vi "CollectCopyrightNotices.vi"() -> ()   [LabVIEW 2020]
uses:
  abd7129a-8e98-49aa-842b-ff99d9e25c9b.vi
panel:
  in  "Folder Path":path
  out "Missing Entires":string[](array[string]) caption="Missing Entires - Anything other than \"pkgconf or vcpkg-*\" needs fixing"
  out "error out":errorcluster
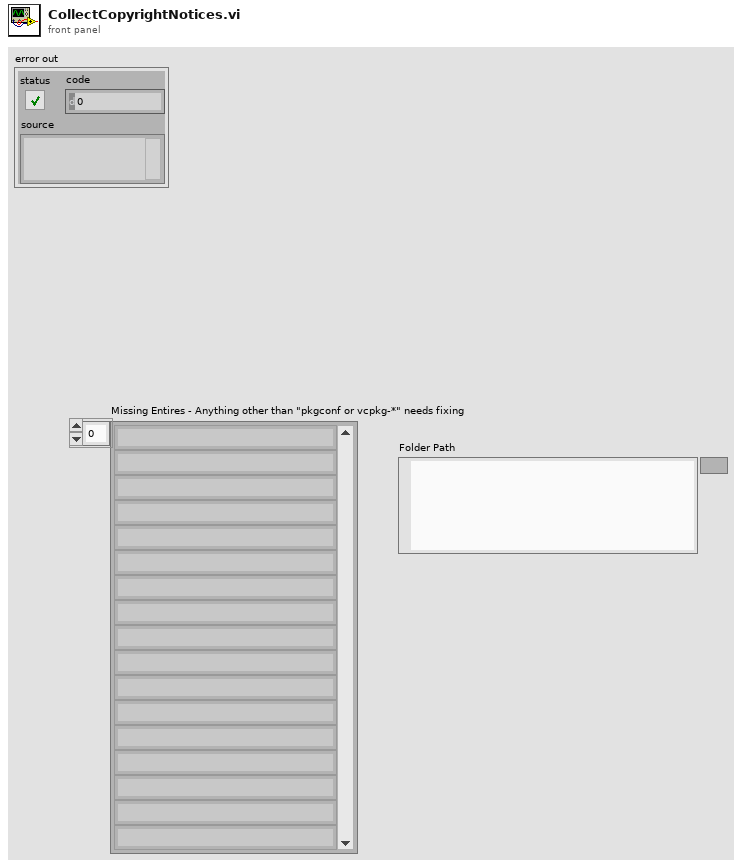
[diagram p1: front panel]
types:
  T1 = enum16{"open", "replace", "create", "open or create", "replace or create", "replace or create with confirmation"}
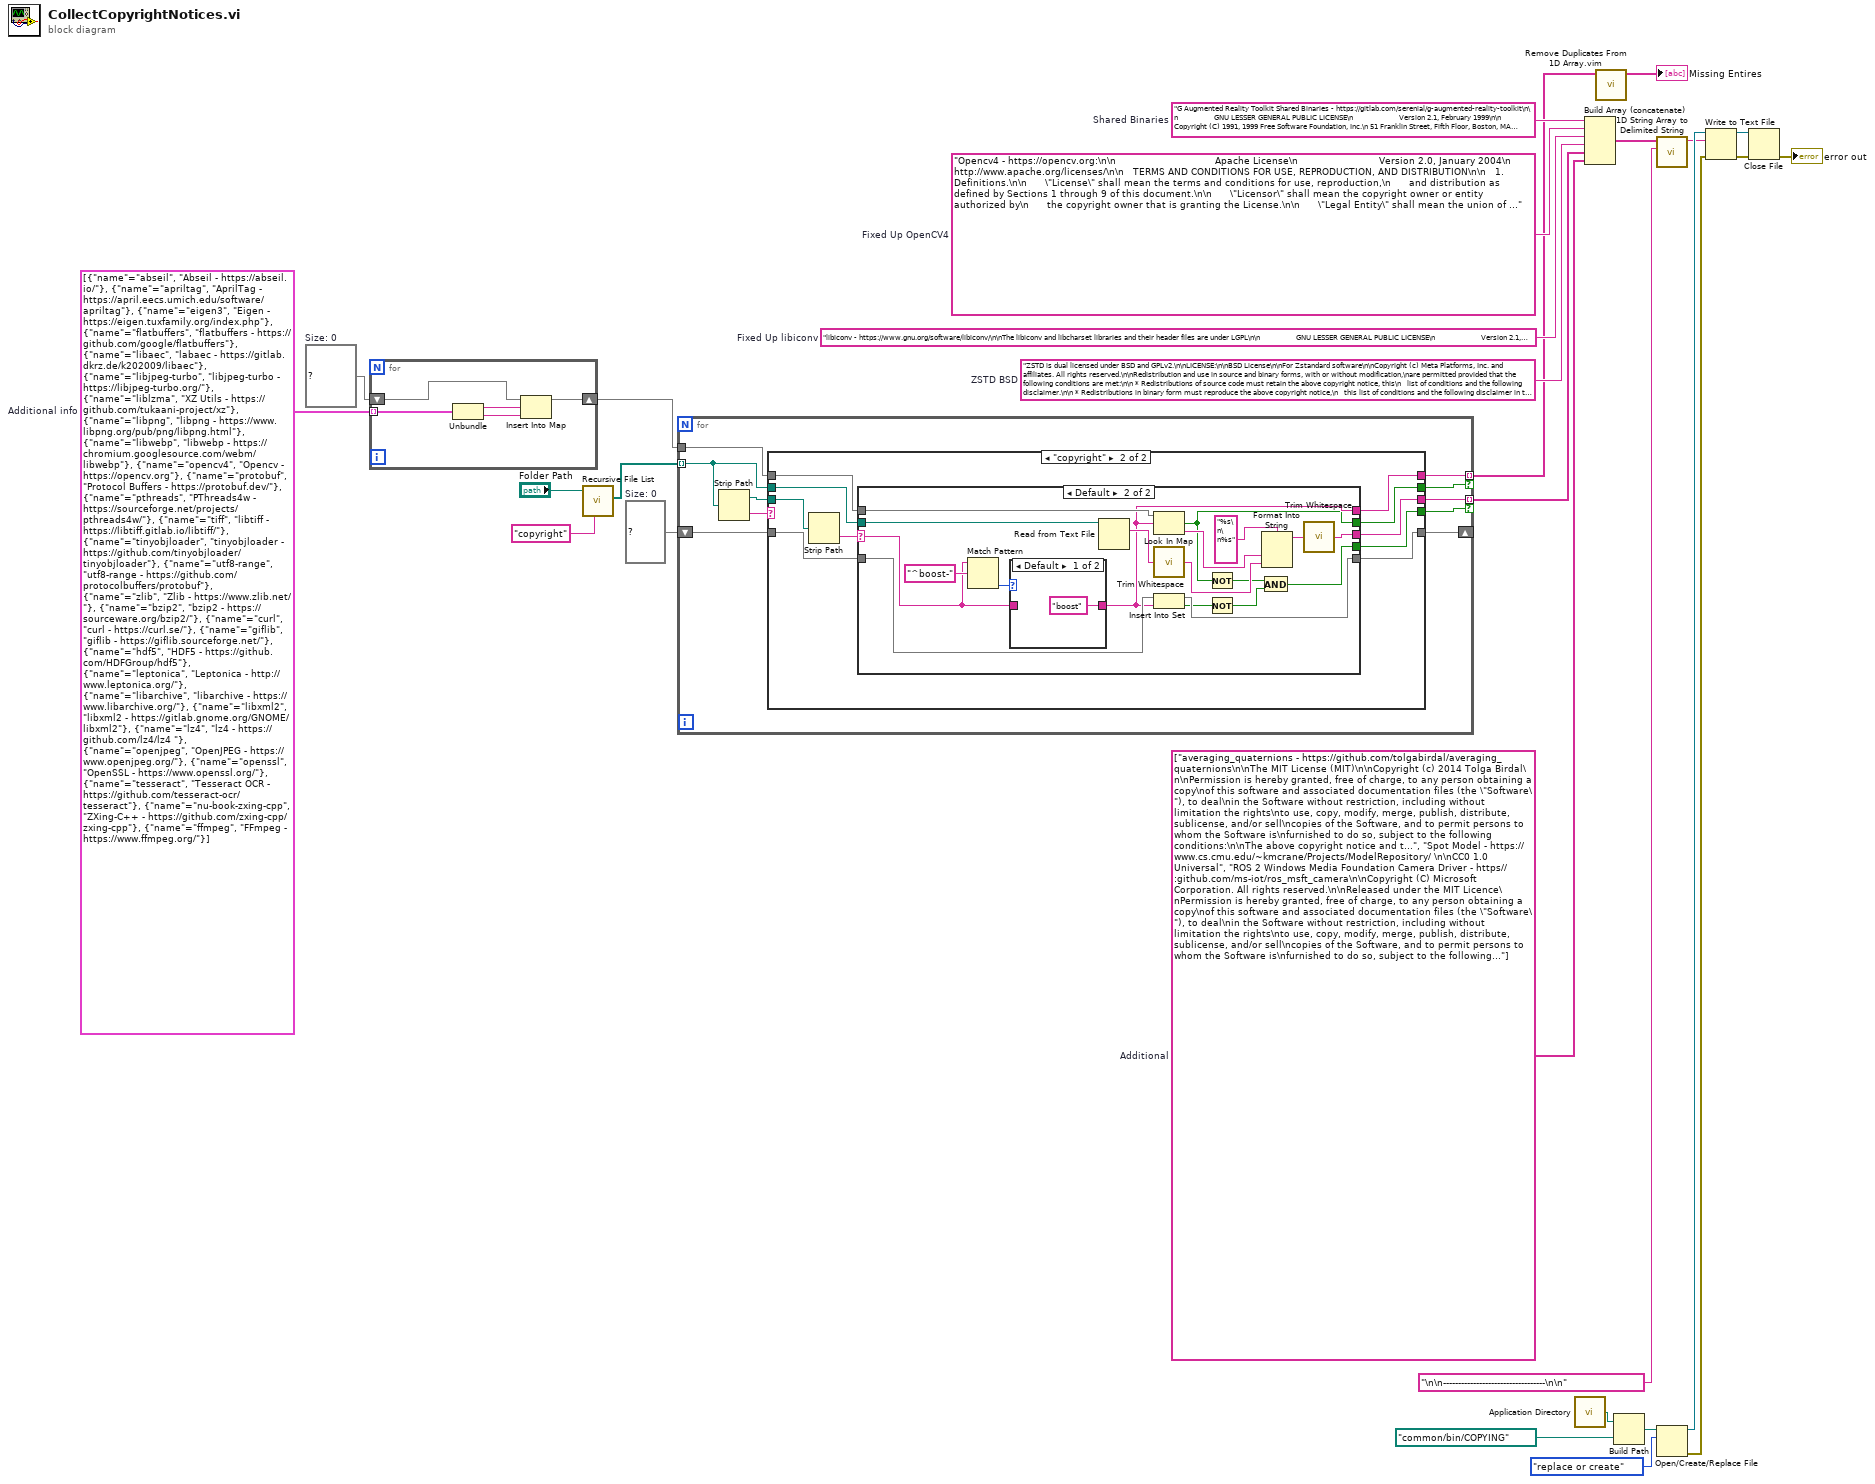
[diagram p0: block diagram]
diagram:
  w4 = "G Augmented Reality Toolkit Shared Binaries - https://gitlab.com/serenial/g-augmented-reality-toolkit\n\n                  GNU LESSER GENERAL PUBLIC LICENSE\n                       Version 2.1, February 1999\n\n Copyright (C) 1991, 1999 Free Software Foundation, Inc.\n 51 Franklin Street, Fifth Floor, Boston, MA  02110-1301  USA\n Everyone is permitted to copy and distribute verbatim copies\n of this license document, but changing it is not allowed.\n\n[This is the first released version of the Lesser GPL.  It also counts\n as the successor of the GNU Library Public License, version 2, hence\n the version number 2.1.]\n\n                            Preamble\n\n  The licenses for most software are designed to take away your\nfreedom to share and change it.  By contrast, the GNU General Public\nLicenses are intended to guarantee your freedom to share and change\nfree software--to make sure the software is free for all its users.\n\n  This license, the Lesser General Public License, applies to some\nspecially designated software packages--typically libraries--of the\nFree Software Foundation and other authors who decide to use it.  You\ncan use it too, but we suggest you first think carefully about whether\nthis license or the ordinary General Public License is the better\nstrategy to use in any particular case, based on the explanations below.\n\n  When we speak of free software, we are referring to freedom of use,\nnot price.  Our General Public Licenses are designed to make sure that\nyou have the freedom to distribute copies of free software (and charge\nfor this service if you wish); that you receive source code or can get\nit if you want it; that you can change the software and use pieces of\nit in new free programs; and that you are informed that you can do\nthese things.\n\n  To protect your rights, we need to make restrictions that forbid\ndistributors to deny you these rights or to ask you to surrender these\nrights.  These restrictions translate to certain responsibilities for\nyou if you distribute copies of the library or if you modify it.\n\n  For example, if you distribute copies of the library, whether gratis\nor for a fee, you must give the recipients all the rights that we gave\nyou.  You must make sure that they, too, receive or can get the source\ncode.  If you link other code with the library, you must provide\ncomplete object files to the recipients, so that they can relink them\nwith the library after making changes to the library and recompiling\nit.  And you must show them these terms so they know their rights.\n\n  We protect your rights with a two-step method: (1) we copyright the\nlibrary, and (2) we offer you this license, which gives you legal\npermission to copy, distribute and/or modify the library.\n\n  To protect each distributor, we want to make it very clear that\nthere is no warranty for the free library.  Also, if the library is\nmodified by someone else and passed on, the recipients should know\nthat what they have is not the original version, so that the original\nauthor's reputation will not be affected by problems that might be\nintroduced by others.\n\n  Finally, software patents pose a constant threat to the existence of\nany free program.  We wish to make sure that a company cannot\neffectively restrict the users of a free program by obtaining a\nrestrictive license from a patent holder.  Therefore, we insist that\nany patent license obtained for a version of the library must be\nconsistent with the full freedom of use specified in this license.\n\n  Most GNU software, including some libraries, is covered by the\nordinary GNU General Public License.  This license, the GNU Lesser\nGeneral Public License, applies to certain designated libraries, and\nis quite different from the ordinary General Public License.  We use\nthis license for certain libraries in order to permit linking those\nlibraries into non-free programs.\n\n  When a program is linked with a library, whether statically or using\na shared library, the combination of the two is legally speaking a\ncombined work, a derivative of the original library.  The ordinary\nGeneral Public License therefore permits such linking only if the\nentire combination fits its criteria of freedom.  The Lesser General\nPublic License permits more lax criteria for linking other code with\nthe library.\n\n  We call this license the \"Lesser\" General Public License because it\ndoes Less to protect the user's freedom than the ordinary General\nPublic License.  It also provides other free software developers Less\nof an advantage over competing non-free programs.  These disadvantages\nare the reason we use the ordinary General Public License for many\nlibraries.  However, the Lesser license provides advantages in certain\nspecial circumstances.\n\n  For example, on rare occasions, there may be a special need to\nencourage the widest possible use of a certain library, so that it becomes\na de-facto standard.  To achieve this, non-free programs must be\nallowed to use the library.  A more frequent case is that a free\nlibrary does the same job as widely used non-free libraries.  In this\ncase, there is little to gain by limiting the free library to free\nsoftware only, so we use the Lesser General Public License.\n\n  In other cases, permission to use a particular library in non-free\nprograms enables a greater number of people to use a large body of\nfree software.  For example, permission to use the GNU C Library in\nnon-free programs enables many more people to use the whole GNU\noperating system, as well as its variant, the GNU/Linux operating\nsystem.\n\n  Although the Lesser General Public License is Less protective of the\nusers' freedom, it does ensure that the user of a program that is\nlinked with the Library has the freedom and the wherewithal to run\nthat program using a modified version of the Library.\n\n  The precise terms and conditions for copying, distribution and\nmodification follow.  Pay close attention to the difference between a\n\"work based on the library\" and a \"work that uses the library\".  The\nformer contains code derived from the library, whereas the latter must\nbe combined with the library in order to run.\n\n                  GNU LESSER GENERAL PUBLIC LICENSE\n   TERMS AND CONDITIONS FOR COPYING, DISTRIBUTION AND MODIFICATION\n\n  0. This License Agreement applies to any software library or other\nprogram which contains a notice placed by the copyright holder or\nother authorized party saying it may be distributed under the terms of\nthis Lesser General Public License (also called \"this License\").\nEach licensee is addressed as \"you\".\n\n  A \"library\" means a collection of software functions and/or data\nprepared so as to be conveniently linked with application programs\n(which use some of those functions and data) to form executables.\n\n  The \"Library\", below, refers to any such software library or work\nwhich has been distributed under these terms.  A \"work based on the\nLibrary\" means either the Library or any derivative work under\ncopyright law: that is to say, a work containing the Library or a\nportion of it, either verbatim or with modifications and/or translated\nstraightforwardly into another language.  (Hereinafter, translation is\nincluded without limitation in the term \"modification\".)\n\n  \"Source code\" for a work means the preferred form of the work for\nmaking modifications to it.  For a library, complete source code means\nall the source code for all modules it contains, plus any associated\ninterface definition files, plus the scripts used to control compilation\nand installation of the library.\n\n  Activities other than copying, distribution and modification are not\ncovered by this License; they are outside its scope.  The act of\nrunning a program using the Library is not restricted, and output from\nsuch a program is covered only if its contents constitute a work based\non the Library (independent of the use of the Library in a tool for\nwriting it).  Whether that is true depends on what the Library does\nand what the program that uses the Library does.\n\n  1. You may copy and distribute verbatim copies of the Library's\ncomplete source code as you receive it, in any medium, provided that\nyou conspicuously and appropriately publish on each copy an\nappropriate copyright notice and disclaimer of warranty; keep intact\nall the notices that refer to this License and to the absence of any\nwarranty; and distribute a copy of this License along with the\nLibrary.\n\n  You may charge a fee for the physical act of transferring a copy,\nand you may at your option offer warranty protection in exchange for a\nfee.\n\n  2. You may modify your copy or copies of the Library or any portion\nof it, thus forming a work based on the Library, and copy and\ndistribute such modifications or work under the terms of Section 1\nabove, provided that you also meet all of these conditions:\n\n    a) The modified work must itself be a software library.\n\n    b) You must cause the files modified to carry prominent notices\n    stating that you changed the files and the date of any change.\n\n    c) You must cause the whole of the work to be licensed at no\n    charge to all third parties under the terms of this License.\n\n    d) If a facility in the modified Library refers to a function or a\n    table of data to be supplied by an application program that uses\n    the facility, other than as an argument passed when the facility\n    is invoked, then you must make a good faith effort to ensure that,\n    in the event an application does not supply such function or\n    table, the facility still operates, and performs whatever part of\n    its purpose remains meaningful.\n\n    (For example, a function in a library to compute square roots has\n    a purpose that is entirely well-defined independent of the\n    application.  Therefore, Subsection 2d requires that any\n    application-supplied function or table used by this function must\n    be optional: if the application does not supply it, the square\n    root function must still compute square roots.)\n\nThese requirements apply to the modified work as a whole.  If\nidentifiable sections of that work are not derived from the Library,\nand can be reasonably considered independent and separate works in\nthemselves, then this License, and its terms, do not apply to those\nsections when you distribute them as separate works.  But when you\ndistribute the same sections as part of a whole which is a work based\non the Library, the distribution of the whole must be on the terms of\nthis License, whose permissions for other licensees extend to the\nentire whole, and thus to each and every part regardless of who wrote\nit.\n\nThus, it is not the intent of this section to claim rights or contest\nyour rights to work written entirely by you; rather, the intent is to\nexercise the right to control the distribution of derivative or\ncollective works based on the Library.\n\nIn addition, mere aggregation of another work not based on the Library\nwith the Library (or with a work based on the Library) on a volume of\na storage or distribution medium does not bring the other work under\nthe scope of this License.\n\n  3. You may opt to apply the terms of the ordinary GNU General Public\nLicense instead of this License to a given copy of the Library.  To do\nthis, you must alter all the notices that refer to this License, so\nthat they refer to the ordinary GNU General Public License, version 2,\ninstead of to this License.  (If a newer version than version 2 of the\nordinary GNU General Public License has appeared, then you can specify\nthat version instead if you wish.)  Do not make any other change in\nthese notices.\n\n  Once this change is made in a given copy, it is irreversible for\nthat copy, so the ordinary GNU General Public License applies to all\nsubsequent copies and derivative works made from that copy.\n\n  This option is useful when you wish to copy part of the code of\nthe Library into a program that is not a library.\n\n  4. You may copy and distribute the Library (or a portion or\nderivative of it, under Section 2) in object code or executable form\nunder the terms of Sections 1 and 2 above provided that you accompany\nit with the complete corresponding machine-readable source code, which\nmust be distributed under the terms of Sections 1 and 2 above on a\nmedium customarily used for software interchange.\n\n  If distribution of object code is made by offering access to copy\nfrom a designated place, then offering equivalent access to copy the\nsource code from the same place satisfies the requirement to\ndistribute the source code, even though third parties are not\ncompelled to copy the source along with the object code.\n\n  5. A program that contains no derivative of any portion of the\nLibrary, but is designed to work with the Library by being compiled or\nlinked with it, is called a \"work that uses the Library\".  Such a\nwork, in isolation, is not a derivative work of the Library, and\ntherefore falls outside the scope of this License.\n\n  However, linking a \"work that uses the Library\" with the Library\ncreates an executable that is a derivative of the Library (because it\ncontains portions of the Library), rather than a \"work that uses the\nlibrary\".  The executable is therefore covered by this License.\nSection 6 states terms for distribution of such executables.\n\n  When a \"work that uses the Library\" uses material from a header file\nthat is part of the Library, the object code for the work may be a\nderivative work of the Library even though the source code is not.\nWhether this is true is especially significant if the work can be\nlinked without the Library, or if the work is itself a library.  The\nthreshold for this to be true is not precisely defined by law.\n\n  If such an object file uses only numerical parameters, data\nstructure layouts and accessors, and small macros and small inline\nfunctions (ten lines or less in length), then the use of the object\nfile is unrestricted, regardless of whether it is legally a derivative\nwork.  (Executables containing this object code plus portions of the\nLibrary will still fall under Section 6.)\n\n  Otherwise, if the work is a derivative of the Library, you may\ndistribute the object code for the work under the terms of Section 6.\nAny executables containing that work also fall under Section 6,\nwhether or not they are linked directly with the Library itself.\n\n  6. As an exception to the Sections above, you may also combine or\nlink a \"work that uses the Library\" with the Library to produce a\nwork containing portions of the Library, and distribute that work\nunder terms of your choice, provided that the terms permit\nmodification of the work for the customer's own use and reverse\nengineering for debugging such modifications.\n\n  You must give prominent notice with each copy of the work that the\nLibrary is used in it and that the Library and its use are covered by\nthis License.  You must supply a copy of this License.  If the work\nduring execution displays copyright notices, you must include the\ncopyright notice for the Library among them, as well as a reference\ndirecting the user to the copy of this License.  Also, you must do one\nof these things:\n\n    a) Accompany the work with the complete corresponding\n    machine-readable source code for the Library including whatever\n    changes were used in the work (which must be distributed under\n    Sections 1 and 2 above); and, if the work is an executable linked\n    with the Library, with the complete machine-readable \"work that\n    uses the Library\", as object code and/or source code, so that the\n    user can modify the Library and then relink to produce a modified\n    executable containing the modified Library.  (It is understood\n    that the user who changes the contents of definitions files in the\n    Library will not necessarily be able to recompile the application\n    to use the modified definitions.)\n\n    b) Use a suitable shared library mechanism for linking with the\n    Library.  A suitable mechanism is one that (1) uses at run time a\n    copy of the library already present on the user's computer system,\n    rather than copying library functions into the executable, and (2)\n    will operate properly with a modified version of the library, if\n    the user installs one, as long as the modified version is\n    interface-compatible with the version that the work was made with.\n\n    c) Accompany the work with a written offer, valid for at\n    least three years, to give the same user the materials\n    specified in Subsection 6a, above, for a charge no more\n    than the cost of performing this distribution.\n\n    d) If distribution of the work is made by offering access to copy\n    from a designated place, offer equivalent access to copy the above\n    specified materials from the same place.\n\n    e) Verify that the user has already received a copy of these\n    materials or that you have already sent this user a copy.\n\n  For an executable, the required form of the \"work that uses the\nLibrary\" must include any data and utility programs needed for\nreproducing the executable from it.  However, as a special exception,\nthe materials to be distributed need not include anything that is\nnormally distributed (in either source or binary form) with the major\ncomponents (compiler, kernel, and so on) of the operating system on\nwhich the executable runs, unless that component itself accompanies\nthe executable.\n\n  It may happen that this requirement contradicts the license\nrestrictions of other proprietary libraries that do not normally\naccompany the operating system.  Such a contradiction means you cannot\nuse both them and the Library together in an executable that you\ndistribute.\n\n  7. You may place library facilities that are a work based on the\nLibrary side-by-side in a single library together with other library\nfacilities not covered by this License, and distribute such a combined\nlibrary, provided that the separate distribution of the work based on\nthe Library and of the other library facilities is otherwise\npermitted, and provided that you do these two things:\n\n    a) Accompany the combined library with a copy of the same work\n    based on the Library, uncombined with any other library\n    facilities.  This must be distributed under the terms of the\n    Sections above.\n\n    b) Give prominent notice with the combined library of the fact\n    that part of it is a work based on the Library, and explaining\n    where to find the accompanying uncombined form of the same work.\n\n  8. You may not copy, modify, sublicense, link with, or distribute\nthe Library except as expressly provided under this License.  Any\nattempt otherwise to copy, modify, sublicense, link with, or\ndistribute the Library is void, and will automatically terminate your\nrights under this License.  However, parties who have received copies,\nor rights, from you under this License will not have their licenses\nterminated so long as such parties remain in full compliance.\n\n  9. You are not required to accept this License, since you have not\nsigned it.  However, nothing else grants you permission to modify or\ndistribute the Library or its derivative works.  These actions are\nprohibited by law if you do not accept this License.  Therefore, by\nmodifying or distributing the Library (or any work based on the\nLibrary), you indicate your acceptance of this License to do so, and\nall its terms and conditions for copying, distributing or modifying\nthe Library or works based on it.\n\n  10. Each time you redistribute the Library (or any work based on the\nLibrary), the recipient automatically receives a license from the\noriginal licensor to copy, distribute, link with or modify the Library\nsubject to these terms and conditions.  You may not impose any further\nrestrictions on the recipients' exercise of the rights granted herein.\nYou are not responsible for enforcing compliance by third parties with\nthis License.\n\n  11. If, as a consequence of a court judgment or allegation of patent\ninfringement or for any other reason (not limited to patent issues),\nconditions are imposed on you (whether by court order, agreement or\notherwise) that contradict the conditions of this License, they do not\nexcuse you from the conditions of this License.  If you cannot\ndistribute so as to satisfy simultaneously your obligations under this\nLicense and any other pertinent obligations, then as a consequence you\nmay not distribute the Library at all.  For example, if a patent\nlicense would not permit royalty-free redistribution of the Library by\nall those who receive copies directly or indirectly through you, then\nthe only way you could satisfy both it and this License would be to\nrefrain entirely from distribution of the Library.\n\nIf any portion of this section is held invalid or unenforceable under any\nparticular circumstance, the balance of the section is intended to apply,\nand the section as a whole is intended to apply in other circumstances.\n\nIt is not the purpose of this section to induce you to infringe any\npatents or other property right claims or to contest validity of any\nsuch claims; this section has the sole purpose of protecting the\nintegrity of the free software distribution system which is\nimplemented by public license practices.  Many people have made\ngenerous contributions to the wide range of software distributed\nthrough that system in reliance on consistent application of that\nsystem; it is up to the author/donor to decide if he or she is willing\nto distribute software through any other system and a licensee cannot\nimpose that choice.\n\nThis section is intended to make thoroughly clear what is believed to\nbe a consequence of the rest of this License.\n\n  12. If the distribution and/or use of the Library is restricted in\ncertain countries either by patents or by copyrighted interfaces, the\noriginal copyright holder who places the Library under this License may add\nan explicit geographical distribution limitation excluding those countries,\nso that distribution is permitted only in or among countries not thus\nexcluded.  In such case, this License incorporates the limitation as if\nwritten in the body of this License.\n\n  13. The Free Software Foundation may publish revised and/or new\nversions of the Lesser General Public License from time to time.\nSuch new versions will be similar in spirit to the present version,\nbut may differ in detail to address new problems or concerns.\n\nEach version is given a distinguishing version number.  If the Library\nspecifies a version number of this License which applies to it and\n\"any later version\", you have the option of following the terms and\nconditions either of that version or of any later version published by\nthe Free Software Foundation.  If the Library does not specify a\nlicense version number, you may choose any version ever published by\nthe Free Software Foundation.\n\n  14. If you wish to incorporate parts of the Library into other free\nprograms whose distribution conditions are incompatible with these,\nwrite to the author to ask for permission.  For software which is\ncopyrighted by the Free Software Foundation, write to the Free\nSoftware Foundation; we sometimes make exceptions for this.  Our\ndecision will be guided by the two goals of preserving the free status\nof all derivatives of our free software and of promoting the sharing\nand reuse of software generally.\n\n                            NO WARRANTY\n\n  15. BECAUSE THE LIBRARY IS LICENSED FREE OF CHARGE, THERE IS NO\nWARRANTY FOR THE LIBRARY, TO THE EXTENT PERMITTED BY APPLICABLE LAW.\nEXCEPT WHEN OTHERWISE STATED IN WRITING THE COPYRIGHT HOLDERS AND/OR\nOTHER PARTIES PROVIDE THE LIBRARY \"AS IS\" WITHOUT WARRANTY OF ANY\nKIND, EITHER EXPRESSED OR IMPLIED, INCLUDING, BUT NOT LIMITED TO, THE\nIMPLIED WARRANTIES OF MERCHANTABILITY AND FITNESS FOR A PARTICULAR\nPURPOSE.  THE ENTIRE RISK AS TO THE QUALITY AND PERFORMANCE OF THE\nLIBRARY IS WITH YOU.  SHOULD THE LIBRARY PROVE DEFECTIVE, YOU ASSUME\nTHE COST OF ALL NECESSARY SERVICING, REPAIR OR CORRECTION.\n\n  16. IN NO EVENT UNLESS REQUIRED BY APPLICABLE LAW OR AGREED TO IN\nWRITING WILL ANY COPYRIGHT HOLDER, OR ANY OTHER PARTY WHO MAY MODIFY\nAND/OR REDISTRIBUTE THE LIBRARY AS PERMITTED ABOVE, BE LIABLE TO YOU\nFOR DAMAGES, INCLUDING ANY GENERAL, SPECIAL, INCIDENTAL OR\nCONSEQUENTIAL DAMAGES ARISING OUT OF THE USE OR INABILITY TO USE THE\nLIBRARY (INCLUDING BUT NOT LIMITED TO LOSS OF DATA OR DATA BEING\nRENDERED INACCURATE OR LOSSES SUSTAINED BY YOU OR THIRD PARTIES OR A\nFAILURE OF THE LIBRARY TO OPERATE WITH ANY OTHER SOFTWARE), EVEN IF\nSUCH HOLDER OR OTHER PARTY HAS BEEN ADVISED OF THE POSSIBILITY OF SUCH\nDAMAGES.\n\n                     END OF TERMS AND CONDITIONS\n\n           How to Apply These Terms to Your New Libraries\n\n  If you develop a new library, and you want it to be of the greatest\npossible use to the public, we recommend making it free software that\neveryone can redistribute and change.  You can do so by permitting\nredistribution under these terms (or, alternatively, under the terms of the\nordinary General Public License).\n\n  To apply these terms, attach the following notices to the library.  It is\nsafest to attach them to the start of each source file to most effectively\nconvey the exclusion of warranty; and each file should have at least the\n\"copyright\" line and a pointer to where the full notice is found.\n\n    <one line to give the library's name and a brief idea of what it does.>\n    Copyright (C) <year>  <name of author>\n\n    This library is free software; you can redistribute it and/or\n    modify it under the terms of the GNU Lesser General Public\n    License as published by the Free Software Foundation; either\n    version 2.1 of the License, or (at your option) any later version.\n\n    This library is distributed in the hope that it will be useful,\n    but WITHOUT ANY WARRANTY; without even the implied warranty of\n    MERCHANTABILITY or FITNESS FOR A PARTICULAR PURPOSE.  See the GNU\n    Lesser General Public License for more details.\n\n    You should have received a copy of the GNU Lesser General Public\n    License along with this library; if not, write to the Free Software\n    Foundation, Inc., 51 Franklin Street, Fifth Floor, Boston, MA  02110-1301\n    USA\n\nAlso add information on how to contact you by electronic and paper mail.\n\nYou should also get your employer (if you work as a programmer) or your\nschool, if any, to sign a \"copyright disclaimer\" for the library, if\nnecessary.  Here is a sample; alter the names:\n\n  Yoyodyne, Inc., hereby disclaims all copyright interest in the\n  library `Frob' (a library for tweaking knobs) written by James Random\n  Hacker.\n\n  <signature of Ty Coon>, 1 April 1990\n  Ty Coon, President of Vice\n\nThat's all there is to it!"  # Shared Binaries
  w5 = set{string} {}  # Size: 0
  w6 = "ZSTD is dual licensed under BSD and GPLv2.\n\nLICENSE:\n\nBSD License\n\nFor Zstandard software\n\nCopyright (c) Meta Platforms, Inc. and affiliates. All rights reserved.\n\nRedistribution and use in source and binary forms, with or without modification,\nare permitted provided that the following conditions are met:\n\n * Redistributions of source code must retain the above copyright notice, this\n   list of conditions and the following disclaimer.\n\n * Redistributions in binary form must reproduce the above copyright notice,\n   this list of conditions and the following disclaimer in the documentation\n   and/or other materials provided with the distribution.\n\n * Neither the name Facebook, nor Meta, nor the names of its contributors may\n   be used to endorse or promote products derived from this software without\n   specific prior written permission.\n\nTHIS SOFTWARE IS PROVIDED BY THE COPYRIGHT HOLDERS AND CONTRIBUTORS \"AS IS\" AND\nANY EXPRESS OR IMPLIED WARRANTIES, INCLUDING, BUT NOT LIMITED TO, THE IMPLIED\nWARRANTIES OF MERCHANTABILITY AND FITNESS FOR A PARTICULAR PURPOSE ARE\nDISCLAIMED. IN NO EVENT SHALL THE COPYRIGHT HOLDER OR CONTRIBUTORS BE LIABLE FOR\nANY DIRECT, INDIRECT, INCIDENTAL, SPECIAL, EXEMPLARY, OR CONSEQUENTIAL DAMAGES\n(INCLUDING, BUT NOT LIMITED TO, PROCUREMENT OF SUBSTITUTE GOODS OR SERVICES;\nLOSS OF USE, DATA, OR PROFITS; OR BUSINESS INTERRUPTION) HOWEVER CAUSED AND ON\nANY THEORY OF LIABILITY, WHETHER IN CONTRACT, STRICT LIABILITY, OR TORT\n(INCLUDING NEGLIGENCE OR OTHERWISE) ARISING IN ANY WAY OUT OF THE USE OF THIS\nSOFTWARE, EVEN IF ADVISED OF THE POSSIBILITY OF SUCH DAMAGE."  # ZSTD BSD
  w7 = "libiconv - https://www.gnu.org/software/libiconv/\n\nThe libiconv and libcharset libraries and their header files are under LGPL\n\n                  GNU LESSER GENERAL PUBLIC LICENSE\n                       Version 2.1, February 1999\n\n Copyright (C) 1991, 1999 Free Software Foundation, Inc.\n 51 Franklin Street, Fifth Floor, Boston, MA  02110-1301  USA\n Everyone is permitted to copy and distribute verbatim copies\n of this license document, but changing it is not allowed.\n\n[This is the first released version of the Lesser GPL.  It also counts\n as the successor of the GNU Library Public License, version 2, hence\n the version number 2.1.]\n\n                            Preamble\n\n  The licenses for most software are designed to take away your\nfreedom to share and change it.  By contrast, the GNU General Public\nLicenses are intended to guarantee your freedom to share and change\nfree software--to make sure the software is free for all its users.\n\n  This license, the Lesser General Public License, applies to some\nspecially designated software packages--typically libraries--of the\nFree Software Foundation and other authors who decide to use it.  You\ncan use it too, but we suggest you first think carefully about whether\nthis license or the ordinary General Public License is the better\nstrategy to use in any particular case, based on the explanations below.\n\n  When we speak of free software, we are referring to freedom of use,\nnot price.  Our General Public Licenses are designed to make sure that\nyou have the freedom to distribute copies of free software (and charge\nfor this service if you wish); that you receive source code or can get\nit if you want it; that you can change the software and use pieces of\nit in new free programs; and that you are informed that you can do\nthese things.\n\n  To protect your rights, we need to make restrictions that forbid\ndistributors to deny you these rights or to ask you to surrender these\nrights.  These restrictions translate to certain responsibilities for\nyou if you distribute copies of the library or if you modify it.\n\n  For example, if you distribute copies of the library, whether gratis\nor for a fee, you must give the recipients all the rights that we gave\nyou.  You must make sure that they, too, receive or can get the source\ncode.  If you link other code with the library, you must provide\ncomplete object files to the recipients, so that they can relink them\nwith the library after making changes to the library and recompiling\nit.  And you must show them these terms so they know their rights.\n\n  We protect your rights with a two-step method: (1) we copyright the\nlibrary, and (2) we offer you this license, which gives you legal\npermission to copy, distribute and/or modify the library.\n\n  To protect each distributor, we want to make it very clear that\nthere is no warranty for the free library.  Also, if the library is\nmodified by someone else and passed on, the recipients should know\nthat what they have is not the original version, so that the original\nauthor's reputation will not be affected by problems that might be\nintroduced by others.\n\f\n  Finally, software patents pose a constant threat to the existence of\nany free program.  We wish to make sure that a company cannot\neffectively restrict the users of a free program by obtaining a\nrestrictive license from a patent holder.  Therefore, we insist that\nany patent license obtained for a version of the library must be\nconsistent with the full freedom of use specified in this license.\n\n  Most GNU software, including some libraries, is covered by the\nordinary GNU General Public License.  This license, the GNU Lesser\nGeneral Public License, applies to certain designated libraries, and\nis quite different from the ordinary General Public License.  We use\nthis license for certain libraries in order to permit linking those\nlibraries into non-free programs.\n\n  When a program is linked with a library, whether statically or using\na shared library, the combination of the two is legally speaking a\ncombined work, a derivative of the original library.  The ordinary\nGeneral Public License therefore permits such linking only if the\nentire combination fits its criteria of freedom.  The Lesser General\nPublic License permits more lax criteria for linking other code with\nthe library.\n\n  We call this license the \"Lesser\" General Public License because it\ndoes Less to protect the user's freedom than the ordinary General\nPublic License.  It also provides other free software developers Less\nof an advantage over competing non-free programs.  These disadvantages\nare the reason we use the ordinary General Public License for many\nlibraries.  However, the Lesser license provides advantages in certain\nspecial circumstances.\n\n  For example, on rare occasions, there may be a special need to\nencourage the widest possible use of a certain library, so that it becomes\na de-facto standard.  To achieve this, non-free programs must be\nallowed to use the library.  A more frequent case is that a free\nlibrary does the same job as widely used non-free libraries.  In this\ncase, there is little to gain by limiting the free library to free\nsoftware only, so we use the Lesser General Public License.\n\n  In other cases, permission to use a particular library in non-free\nprograms enables a greater number of people to use a large body of\nfree software.  For example, permission to use the GNU C Library in\nnon-free programs enables many more people to use the whole GNU\noperating system, as well as its variant, the GNU/Linux operating\nsystem.\n\n  Although the Lesser General Public License is Less protective of the\nusers' freedom, it does ensure that the user of a program that is\nlinked with the Library has the freedom and the wherewithal to run\nthat program using a modified version of the Library.\n\n  The precise terms and conditions for copying, distribution and\nmodification follow.  Pay close attention to the difference between a\n\"work based on the library\" and a \"work that uses the library\".  The\nformer contains code derived from the library, whereas the latter must\nbe combined with the library in order to run.\n\n                  GNU LESSER GENERAL PUBLIC LICENSE\n   TERMS AND CONDITIONS FOR COPYING, DISTRIBUTION AND MODIFICATION\n\n  0. This License Agreement applies to any software library or other\nprogram which contains a notice placed by the copyright holder or\nother authorized party saying it may be distributed under the terms of\nthis Lesser General Public License (also called \"this License\").\nEach licensee is addressed as \"you\".\n\n  A \"library\" means a collection of software functions and/or data\nprepared so as to be conveniently linked with application programs\n(which use some of those functions and data) to form executables.\n\n  The \"Library\", below, refers to any such software library or work\nwhich has been distributed under these terms.  A \"work based on the\nLibrary\" means either the Library or any derivative work under\ncopyright law: that is to say, a work containing the Library or a\nportion of it, either verbatim or with modifications and/or translated\nstraightforwardly into another language.  (Hereinafter, translation is\nincluded without limitation in the term \"modification\".)\n\n  \"Source code\" for a work means the preferred form of the work for\nmaking modifications to it.  For a library, complete source code means\nall the source code for all modules it contains, plus any associated\ninterface definition files, plus the scripts used to control compilation\nand installation of the library.\n\n  Activities other than copying, distribution and modification are not\ncovered by this License; they are outside its scope.  The act of\nrunning a program using the Library is not restricted, and output from\nsuch a program is covered only if its contents constitute a work based\non the Library (independent of the use of the Library in a tool for\nwriting it).  Whether that is true depends on what the Library does\nand what the program that uses the Library does.\n\n  1. You may copy and distribute verbatim copies of the Library's\ncomplete source code as you receive it, in any medium, provided that\nyou conspicuously and appropriately publish on each copy an\nappropriate copyright notice and disclaimer of warranty; keep intact\nall the notices that refer to this License and to the absence of any\nwarranty; and distribute a copy of this License along with the\nLibrary.\n\n  You may charge a fee for the physical act of transferring a copy,\nand you may at your option offer warranty protection in exchange for a\nfee.\n\n  2. You may modify your copy or copies of the Library or any portion\nof it, thus forming a work based on the Library, and copy and\ndistribute such modifications or work under the terms of Section 1\nabove, provided that you also meet all of these conditions:\n\n    a) The modified work must itself be a software library.\n\n    b) You must cause the files modified to carry prominent notices\n    stating that you changed the files and the date of any change.\n\n    c) You must cause the whole of the work to be licensed at no\n    charge to all third parties under the terms of this License.\n\n    d) If a facility in the modified Library refers to a function or a\n    table of data to be supplied by an application program that uses\n    the facility, other than as an argument passed when the facility\n    is invoked, then you must make a good faith effort to ensure that,\n    in the event an application does not supply such function or\n    table, the facility still operates, and performs whatever part of\n    its purpose remains meaningful.\n\n    (For example, a function in a library to compute square roots has\n    a purpose that is entirely well-defined independent of the\n    application.  Therefore, Subsection 2d requires that any\n    application-supplied function or table used by this function must\n    be optional: if the application does not supply it, the square\n    root function must still compute square roots.)\n\nThese requirements apply to the modified work as a whole.  If\nidentifiable sections of that work are not derived from the Library,\nand can be reasonably considered independent and separate works in\nthemselves, then this License, and its terms, do not apply to those\nsections when you distribute them as separate works.  But when you\ndistribute the same sections as part of a whole which is a work based\non the Library, the distribution of the whole must be on the terms of\nthis License, whose permissions for other licensees extend to the\nentire whole, and thus to each and every part regardless of who wrote\nit.\n\nThus, it is not the intent of this section to claim rights or contest\nyour rights to work written entirely by you; rather, the intent is to\nexercise the right to control the distribution of derivative or\ncollective works based on the Library.\n\nIn addition, mere aggregation of another work not based on the Library\nwith the Library (or with a work based on the Library) on a volume of\na storage or distribution medium does not bring the other work under\nthe scope of this License.\n\n  3. You may opt to apply the terms of the ordinary GNU General Public\nLicense instead of this License to a given copy of the Library.  To do\nthis, you must alter all the notices that refer to this License, so\nthat they refer to the ordinary GNU General Public License, version 2,\ninstead of to this License.  (If a newer version than version 2 of the\nordinary GNU General Public License has appeared, then you can specify\nthat version instead if you wish.)  Do not make any other change in\nthese notices.\n\n  Once this change is made in a given copy, it is irreversible for\nthat copy, so the ordinary GNU General Public License applies to all\nsubsequent copies and derivative works made from that copy.\n\n  This option is useful when you wish to copy part of the code of\nthe Library into a program that is not a library.\n\n  4. You may copy and distribute the Library (or a portion or\nderivative of it, under Section 2) in object code or executable form\nunder the terms of Sections 1 and 2 above provided that you accompany\nit with the complete corresponding machine-readable source code, which\nmust be distributed under the terms of Sections 1 and 2 above on a\nmedium customarily used for software interchange.\n\n  If distribution of object code is made by offering access to copy\nfrom a designated place, then offering equivalent access to copy the\nsource code from the same place satisfies the requirement to\ndistribute the source code, even though third parties are not\ncompelled to copy the source along with the object code.\n\n  5. A program that contains no derivative of any portion of the\nLibrary, but is designed to work with the Library by being compiled or\nlinked with it, is called a \"work that uses the Library\".  Such a\nwork, in isolation, is not a derivative work of the Library, and\ntherefore falls outside the scope of this License.\n\n  However, linking a \"work that uses the Library\" with the Library\ncreates an executable that is a derivative of the Library (because it\ncontains portions of the Library), rather than a \"work that uses the\nlibrary\".  The executable is therefore covered by this License.\nSection 6 states terms for distribution of such executables.\n\n  When a \"work that uses the Library\" uses material from a header file\nthat is part of the Library, the object code for the work may be a\nderivative work of the Library even though the source code is not.\nWhether this is true is especially significant if the work can be\nlinked without the Library, or if the work is itself a library.  The\nthreshold for this to be true is not precisely defined by law.\n\n  If such an object file uses only numerical parameters, data\nstructure layouts and accessors, and small macros and small inline\nfunctions (ten lines or less in length), then the use of the object\nfile is unrestricted, regardless of whether it is legally a derivative\nwork.  (Executables containing this object code plus portions of the\nLibrary will still fall under Section 6.)\n\n  Otherwise, if the work is a derivative of the Library, you may\ndistribute the object code for the work under the terms of Section 6.\nAny executables containing that work also fall under Section 6,\nwhether or not they are linked directly with the Library itself.\n\n  6. As an exception to the Sections above, you may also combine or\nlink a \"work that uses the Library\" with the Library to produce a\nwork containing portions of the Library, and distribute that work\nunder terms of your choice, provided that the terms permit\nmodification of the work for the customer's own use and reverse\nengineering for debugging such modifications.\n\n  You must give prominent notice with each copy of the work that the\nLibrary is used in it and that the Library and its use are covered by\nthis License.  You must supply a copy of this License.  If the work\nduring execution displays copyright notices, you must include the\ncopyright notice for the Library among them, as well as a reference\ndirecting the user to the copy of this License.  Also, you must do one\nof these things:\n\n    a) Accompany the work with the complete corresponding\n    machine-readable source code for the Library including whatever\n    changes were used in the work (which must be distributed under\n    Sections 1 and 2 above); and, if the work is an executable linked\n    with the Library, with the complete machine-readable \"work that\n    uses the Library\", as object code and/or source code, so that the\n    user can modify the Library and then relink to produce a modified\n    executable containing the modified Library.  (It is understood\n    that the user who changes the contents of definitions files in the\n    Library will not necessarily be able to recompile the application\n    to use the modified definitions.)\n\n    b) Use a suitable shared library mechanism for linking with the\n    Library.  A suitable mechanism is one that (1) uses at run time a\n    copy of the library already present on the user's computer system,\n    rather than copying library functions into the executable, and (2)\n    will operate properly with a modified version of the library, if\n    the user installs one, as long as the modified version is\n    interface-compatible with the version that the work was made with.\n\n    c) Accompany the work with a written offer, valid for at\n    least three years, to give the same user the materials\n    specified in Subsection 6a, above, for a charge no more\n    than the cost of performing this distribution.\n\n    d) If distribution of the work is made by offering access to copy\n    from a designated place, offer equivalent access to copy the above\n    specified materials from the same place.\n\n    e) Verify that the user has already received a copy of these\n    materials or that you have already sent this user a copy.\n\n  For an executable, the required form of the \"work that uses the\nLibrary\" must include any data and utility programs needed for\nreproducing the executable from it.  However, as a special exception,\nthe materials to be distributed need not include anything that is\nnormally distributed (in either source or binary form) with the major\ncomponents (compiler, kernel, and so on) of the operating system on\nwhich the executable runs, unless that component itself accompanies\nthe executable.\n\n  It may happen that this requirement contradicts the license\nrestrictions of other proprietary libraries that do not normally\naccompany the operating system.  Such a contradiction means you cannot\nuse both them and the Library together in an executable that you\ndistribute.\n\n  7. You may place library facilities that are a work based on the\nLibrary side-by-side in a single library together with other library\nfacilities not covered by this License, and distribute such a combined\nlibrary, provided that the separate distribution of the work based on\nthe Library and of the other library facilities is otherwise\npermitted, and provided that you do these two things:\n\n    a) Accompany the combined library with a copy of the same work\n    based on the Library, uncombined with any other library\n    facilities.  This must be distributed under the terms of the\n    Sections above.\n\n    b) Give prominent notice with the combined library of the fact\n    that part of it is a work based on the Library, and explaining\n    where to find the accompanying uncombined form of the same work.\n\n  8. You may not copy, modify, sublicense, link with, or distribute\nthe Library except as expressly provided under this License.  Any\nattempt otherwise to copy, modify, sublicense, link with, or\ndistribute the Library is void, and will automatically terminate your\nrights under this License.  However, parties who have received copies,\nor rights, from you under this License will not have their licenses\nterminated so long as such parties remain in full compliance.\n\n  9. You are not required to accept this License, since you have not\nsigned it.  However, nothing else grants you permission to modify or\ndistribute the Library or its derivative works.  These actions are\nprohibited by law if you do not accept this License.  Therefore, by\nmodifying or distributing the Library (or any work based on the\nLibrary), you indicate your acceptance of this License to do so, and\nall its terms and conditions for copying, distributing or modifying\nthe Library or works based on it.\n\n  10. Each time you redistribute the Library (or any work based on the\nLibrary), the recipient automatically receives a license from the\noriginal licensor to copy, distribute, link with or modify the Library\nsubject to these terms and conditions.  You may not impose any further\nrestrictions on the recipients' exercise of the rights granted herein.\nYou are not responsible for enforcing compliance by third parties with\nthis License.\n\n  11. If, as a consequence of a court judgment or allegation of patent\ninfringement or for any other reason (not limited to patent issues),\nconditions are imposed on you (whether by court order, agreement or\notherwise) that contradict the conditions of this License, they do not\nexcuse you from the conditions of this License.  If you cannot\ndistribute so as to satisfy simultaneously your obligations under this\nLicense and any other pertinent obligations, then as a consequence you\nmay not distribute the Library at all.  For example, if a patent\nlicense would not permit royalty-free redistribution of the Library by\nall those who receive copies directly or indirectly through you, then\nthe only way you could satisfy both it and this License would be to\nrefrain entirely from distribution of the Library.\n\nIf any portion of this section is held invalid or unenforceable under any\nparticular circumstance, the balance of the section is intended to apply,\nand the section as a whole is intended to apply in other circumstances.\n\nIt is not the purpose of this section to induce you to infringe any\npatents or other property right claims or to contest validity of any\nsuch claims; this section has the sole purpose of protecting the\nintegrity of the free software distribution system which is\nimplemented by public license practices.  Many people have made\ngenerous contributions to the wide range of software distributed\nthrough that system in reliance on consistent application of that\nsystem; it is up to the author/donor to decide if he or she is willing\nto distribute software through any other system and a licensee cannot\nimpose that choice.\n\nThis section is intended to make thoroughly clear what is believed to\nbe a consequence of the rest of this License.\n\n  12. If the distribution and/or use of the Library is restricted in\ncertain countries either by patents or by copyrighted interfaces, the\noriginal copyright holder who places the Library under this License may add\nan explicit geographical distribution limitation excluding those countries,\nso that distribution is permitted only in or among countries not thus\nexcluded.  In such case, this License incorporates the limitation as if\nwritten in the body of this License.\n\n  13. The Free Software Foundation may publish revised and/or new\nversions of the Lesser General Public License from time to time.\nSuch new versions will be similar in spirit to the present version,\nbut may differ in detail to address new problems or concerns.\n\nEach version is given a distinguishing version number.  If the Library\nspecifies a version number of this License which applies to it and\n\"any later version\", you have the option of following the terms and\nconditions either of that version or of any later version published by\nthe Free Software Foundation.  If the Library does not specify a\nlicense version number, you may choose any version ever published by\nthe Free Software Foundation.\n\n  14. If you wish to incorporate parts of the Library into other free\nprograms whose distribution conditions are incompatible with these,\nwrite to the author to ask for permission.  For software which is\ncopyrighted by the Free Software Foundation, write to the Free\nSoftware Foundation; we sometimes make exceptions for this.  Our\ndecision will be guided by the two goals of preserving the free status\nof all derivatives of our free software and of promoting the sharing\nand reuse of software generally.\n\n                            NO WARRANTY\n\n  15. BECAUSE THE LIBRARY IS LICENSED FREE OF CHARGE, THERE IS NO\nWARRANTY FOR THE LIBRARY, TO THE EXTENT PERMITTED BY APPLICABLE LAW.\nEXCEPT WHEN OTHERWISE STATED IN WRITING THE COPYRIGHT HOLDERS AND/OR\nOTHER PARTIES PROVIDE THE LIBRARY \"AS IS\" WITHOUT WARRANTY OF ANY\nKIND, EITHER EXPRESSED OR IMPLIED, INCLUDING, BUT NOT LIMITED TO, THE\nIMPLIED WARRANTIES OF MERCHANTABILITY AND FITNESS FOR A PARTICULAR\nPURPOSE.  THE ENTIRE RISK AS TO THE QUALITY AND PERFORMANCE OF THE\nLIBRARY IS WITH YOU.  SHOULD THE LIBRARY PROVE DEFECTIVE, YOU ASSUME\nTHE COST OF ALL NECESSARY SERVICING, REPAIR OR CORRECTION.\n\n  16. IN NO EVENT UNLESS REQUIRED BY APPLICABLE LAW OR AGREED TO IN\nWRITING WILL ANY COPYRIGHT HOLDER, OR ANY OTHER PARTY WHO MAY MODIFY\nAND/OR REDISTRIBUTE THE LIBRARY AS PERMITTED ABOVE, BE LIABLE TO YOU\nFOR DAMAGES, INCLUDING ANY GENERAL, SPECIAL, INCIDENTAL OR\nCONSEQUENTIAL DAMAGES ARISING OUT OF THE USE OR INABILITY TO USE THE\nLIBRARY (INCLUDING BUT NOT LIMITED TO LOSS OF DATA OR DATA BEING\nRENDERED INACCURATE OR LOSSES SUSTAINED BY YOU OR THIRD PARTIES OR A\nFAILURE OF THE LIBRARY TO OPERATE WITH ANY OTHER SOFTWARE), EVEN IF\nSUCH HOLDER OR OTHER PARTY HAS BEEN ADVISED OF THE POSSIBILITY OF SUCH\nDAMAGES.\n\n                     END OF TERMS AND CONDITIONS"  # Fixed Up libiconv
  w20 = "Opencv4 - https://opencv.org:\n\n                                 Apache License\n                           Version 2.0, January 2004\n                        http://www.apache.org/licenses/\n\n   TERMS AND CONDITIONS FOR USE, REPRODUCTION, AND DISTRIBUTION\n\n   1. Definitions.\n\n      \"License\" shall mean the terms and conditions for use, reproduction,\n      and distribution as defined by Sections 1 through 9 of this document.\n\n      \"Licensor\" shall mean the copyright owner or entity authorized by\n      the copyright owner that is granting the License.\n\n      \"Legal Entity\" shall mean the union of the acting entity and all\n      other entities that control, are controlled by, or are under common\n      control with that entity. For the purposes of this definition,\n      \"control\" means (i) the power, direct or indirect, to cause the\n      direction or management of such entity, whether by contract or\n      otherwise, or (ii) ownership of fifty percent (50%) or more of the\n      outstanding shares, or (iii) beneficial ownership of such entity.\n\n      \"You\" (or \"Your\") shall mean an individual or Legal Entity\n      exercising permissions granted by this License.\n\n      \"Source\" form shall mean the preferred form for making modifications,\n      including but not limited to software source code, documentation\n      source, and configuration files.\n\n      \"Object\" form shall mean any form resulting from mechanical\n      transformation or translation of a Source form, including but\n      not limited to compiled object code, generated documentation,\n      and conversions to other media types.\n\n      \"Work\" shall mean the work of authorship, whether in Source or\n      Object form, made available under the License, as indicated by a\n      copyright notice that is included in or attached to the work\n      (an example is provided in the Appendix below).\n\n      \"Derivative Works\" shall mean any work, whether in Source or Object\n      form, that is based on (or derived from) the Work and for which the\n      editorial revisions, annotations, elaborations, or other modifications\n      represent, as a whole, an original work of authorship. For the purposes\n      of this License, Derivative Works shall not include works that remain\n      separable from, or merely link (or bind by name) to the interfaces of,\n      the Work and Derivative Works thereof.\n\n      \"Contribution\" shall mean any work of authorship, including\n      the original version of the Work and any modifications or additions\n      to that Work or Derivative Works thereof, that is intentionally\n      submitted to Licensor for inclusion in the Work by the copyright owner\n      or by an individual or Legal Entity authorized to submit on behalf of\n      the copyright owner. For the purposes of this definition, \"submitted\"\n      means any form of electronic, verbal, or written communication sent\n      to the Licensor or its representatives, including but not limited to\n      communication on electronic mailing lists, source code control systems,\n      and issue tracking systems that are managed by, or on behalf of, the\n      Licensor for the purpose of discussing and improving the Work, but\n      excluding communication that is conspicuously marked or otherwise\n      designated in writing by the copyright owner as \"Not a Contribution.\"\n\n      \"Contributor\" shall mean Licensor and any individual or Legal Entity\n      on behalf of whom a Contribution has been received by Licensor and\n      subsequently incorporated within the Work.\n\n   2. Grant of Copyright License. Subject to the terms and conditions of\n      this License, each Contributor hereby grants to You a perpetual,\n      worldwide, non-exclusive, no-charge, royalty-free, irrevocable\n      copyright license to reproduce, prepare Derivative Works of,\n      publicly display, publicly perform, sublicense, and distribute the\n      Work and such Derivative Works in Source or Object form.\n\n   3. Grant of Patent License. Subject to the terms and conditions of\n      this License, each Contributor hereby grants to You a perpetual,\n      worldwide, non-exclusive, no-charge, royalty-free, irrevocable\n      (except as stated in this section) patent license to make, have made,\n      use, offer to sell, sell, import, and otherwise transfer the Work,\n      where such license applies only to those patent claims licensable\n      by such Contributor that are necessarily infringed by their\n      Contribution(s) alone or by combination of their Contribution(s)\n      with the Work to which such Contribution(s) was submitted. If You\n      institute patent litigation against any entity (including a\n      cross-claim or counterclaim in a lawsuit) alleging that the Work\n      or a Contribution incorporated within the Work constitutes direct\n      or contributory patent infringement, then any patent licenses\n      granted to You under this License for that Work shall terminate\n      as of the date such litigation is filed.\n\n   4. Redistribution. You may reproduce and distribute copies of the\n      Work or Derivative Works thereof in any medium, with or without\n      modifications, and in Source or Object form, provided that You\n      meet the following conditions:\n\n      (a) You must give any other recipients of the Work or\n          Derivative Works a copy of this License; and\n\n      (b) You must cause any modified files to carry prominent notices\n          stating that You changed the files; and\n\n      (c) You must retain, in the Source form of any Derivative Works\n          that You distribute, all copyright, patent, trademark, and\n          attribution notices from the Source form of the Work,\n          excluding those notices that do not pertain to any part of\n          the Derivative Works; and\n\n      (d) If the Work includes a \"NOTICE\" text file as part of its\n          distribution, then any Derivative Works that You distribute must\n          include a readable copy of the attribution notices contained\n          within such NOTICE file, excluding those notices that do not\n          pertain to any part of the Derivative Works, in at least one\n          of the following places: within a NOTICE text file distributed\n          as part of the Derivative Works; within the Source form or\n          documentation, if provided along with the Derivative Works; or,\n          within a display generated by the Derivative Works, if and\n          wherever such third-party notices normally appear. The contents\n          of the NOTICE file are for informational purposes only and\n          do not modify the License. You may add Your own attribution\n          notices within Derivative Works that You distribute, alongside\n          or as an addendum to the NOTICE text from the Work, provided\n          that such additional attribution notices cannot be construed\n          as modifying the License.\n\n      You may add Your own copyright statement to Your modifications and\n      may provide additional or different license terms and conditions\n      for use, reproduction, or distribution of Your modifications, or\n      for any such Derivative Works as a whole, provided Your use,\n      reproduction, and distribution of the Work otherwise complies with\n      the conditions stated in this License.\n\n   5. Submission of Contributions. Unless You explicitly state otherwise,\n      any Contribution intentionally submitted for inclusion in the Work\n      by You to the Licensor shall be under the terms and conditions of\n      this License, without any additional terms or conditions.\n      Notwithstanding the above, nothing herein shall supersede or modify\n      the terms of any separate license agreement you may have executed\n      with Licensor regarding such Contributions.\n\n   6. Trademarks. This License does not grant permission to use the trade\n      names, trademarks, service marks, or product names of the Licensor,\n      except as required for reasonable and customary use in describing the\n      origin of the Work and reproducing the content of the NOTICE file.\n\n   7. Disclaimer of Warranty. Unless required by applicable law or\n      agreed to in writing, Licensor provides the Work (and each\n      Contributor provides its Contributions) on an \"AS IS\" BASIS,\n      WITHOUT WARRANTIES OR CONDITIONS OF ANY KIND, either express or\n      implied, including, without limitation, any warranties or conditions\n      of TITLE, NON-INFRINGEMENT, MERCHANTABILITY, or FITNESS FOR A\n      PARTICULAR PURPOSE. You are solely responsible for determining the\n      appropriateness of using or redistributing the Work and assume any\n      risks associated with Your exercise of permissions under this License.\n\n   8. Limitation of Liability. In no event and under no legal theory,\n      whether in tort (including negligence), contract, or otherwise,\n      unless required by applicable law (such as deliberate and grossly\n      negligent acts) or agreed to in writing, shall any Contributor be\n      liable to You for damages, including any direct, indirect, special,\n      incidental, or consequential damages of any character arising as a\n      result of this License or out of the use or inability to use the\n      Work (including but not limited to damages for loss of goodwill,\n      work stoppage, computer failure or malfunction, or any and all\n      other commercial damages or losses), even if such Contributor\n      has been advised of the possibility of such damages.\n\n   9. Accepting Warranty or Additional Liability. While redistributing\n      the Work or Derivative Works thereof, You may choose to offer,\n      and charge a fee for, acceptance of support, warranty, indemnity,\n      or other liability obligations and/or rights consistent with this\n      License. However, in accepting such obligations, You may act only\n      on Your own behalf and on Your sole responsibility, not on behalf\n      of any other Contributor, and only if You agree to indemnify,\n      defend, and hold each Contributor harmless for any liability\n      incurred by, or claims asserted against, such Contributor by reason\n      of your accepting any such warranty or additional liability.\n\n   END OF TERMS AND CONDITIONS\n\n   APPENDIX: How to apply the Apache License to your work.\n\n      To apply the Apache License to your work, attach the following\n      boilerplate notice, with the fields enclosed by brackets \"[]\"\n      replaced with your own identifying information. (Don't include\n      the brackets!)  The text should be enclosed in the appropriate\n      comment syntax for the file format. We also recommend that a\n      file or class name and description of purpose be included on the\n      same \"printed page\" as the copyright notice for easier\n      identification within third-party archives.\n\n   Copyright [yyyy] [name of copyright owner]\n\n   Licensed under the Apache License, Version 2.0 (the \"License\");\n   you may not use this file except in compliance with the License.\n   You may obtain a copy of the License at\n\n       http://www.apache.org/licenses/LICENSE-2.0\n\n   Unless required by applicable law or agreed to in writing, software\n   distributed under the License is distributed on an \"AS IS\" BASIS,\n   WITHOUT WARRANTIES OR CONDITIONS OF ANY KIND, either express or implied.\n   See the License for the specific language governing permissions and\n   limitations under the License.\n\n\nSoftFloat-COPYING.txt:\n\nLicense for Berkeley SoftFloat Release 3c\n\nJohn R. Hauser\n2017 February 10\n\nThe following applies to the whole of SoftFloat Release 3c as well as to\neach source file individually.\n\nCopyright 2011, 2012, 2013, 2014, 2015, 2016, 2017 The Regents of the\nUniversity of California.  All rights reserved.\n\nRedistribution and use in source and binary forms, with or without\nmodification, are permitted provided that the following conditions are met:\n\n 1. Redistributions of source code must retain the above copyright notice,\n    this list of conditions, and the following disclaimer.\n\n 2. Redistributions in binary form must reproduce the above copyright\n    notice, this list of conditions, and the following disclaimer in the\n    documentation and/or other materials provided with the distribution.\n\n 3. Neither the name of the University nor the names of its contributors\n    may be used to endorse or promote products derived from this software\n    without specific prior written permission.\n\nTHIS SOFTWARE IS PROVIDED BY THE REGENTS AND CONTRIBUTORS \"AS IS\", AND ANY\nEXPRESS OR IMPLIED WARRANTIES, INCLUDING, BUT NOT LIMITED TO, THE IMPLIED\nWARRANTIES OF MERCHANTABILITY AND FITNESS FOR A PARTICULAR PURPOSE, ARE\nDISCLAIMED.  IN NO EVENT SHALL THE REGENTS OR CONTRIBUTORS BE LIABLE FOR ANY\nDIRECT, INDIRECT, INCIDENTAL, SPECIAL, EXEMPLARY, OR CONSEQUENTIAL DAMAGES\n(INCLUDING, BUT NOT LIMITED TO, PROCUREMENT OF SUBSTITUTE GOODS OR SERVICES;\nLOSS OF USE, DATA, OR PROFITS; OR BUSINESS INTERRUPTION) HOWEVER CAUSED AND\nON ANY THEORY OF LIABILITY, WHETHER IN CONTRACT, STRICT LIABILITY, OR TORT\n(INCLUDING NEGLIGENCE OR OTHERWISE) ARISING IN ANY WAY OUT OF THE USE OF\nTHIS SOFTWARE, EVEN IF ADVISED OF THE POSSIBILITY OF SUCH DAMAGE.\n\nIntel Simplified Software License (Version October 2022)\n\nIntel(R) Integrated Performance Primitives (Intel(R) IPP) : Copyright (C) 1997 Intel Corporation\n\nUse and Redistribution. You may use and redistribute the software, which is\nprovided in binary form only, (the \"Software\"), without modification,\nprovided the following conditions are met:\n\n* Redistributions must reproduce the above copyright notice and these\n  terms of use in the Software and in the documentation and/or other materials\n  provided with the distribution.\n* Neither the name of Intel nor the names of its suppliers may be used to\n  endorse or promote products derived from this Software without specific\n  prior written permission.\n* No reverse engineering, decompilation, or disassembly of the Software is\n  permitted, nor any modification or alteration of the Software or its operation\n  at any time, including during execution.\n\nNo other licenses. Except as provided in the preceding section, Intel grants no\nlicenses or other rights by implication, estoppel or otherwise to, patent,\ncopyright, trademark, trade name, service mark or other intellectual property\nlicenses or rights of Intel.\n\nThird party software.  \"Third Party Software\" means the files (if any) listed\nin the \"third-party-software.txt\" or other similarly-named text file that may\nbe included with the Software. Third Party Software, even if included with the\ndistribution of the Software, may be governed by separate license terms, including\nwithout limitation, third party license terms, open source software notices and\nterms, and/or other Intel software license terms. These separate license terms\nsolely govern Your use of the Third Party Software.\n\nDISCLAIMER. THIS SOFTWARE IS PROVIDED \"AS IS\" AND ANY EXPRESS OR IMPLIED\nWARRANTIES, INCLUDING, BUT NOT LIMITED TO, THE IMPLIED WARRANTIES OF\nMERCHANTABILITY, FITNESS FOR A PARTICULAR PURPOSE, AND NON-INFRINGEMENT ARE\nDISCLAIMED. THIS SOFTWARE IS NOT INTENDED FOR USE IN SYSTEMS OR APPLICATIONS\nWHERE FAILURE OF THE SOFTWARE MAY CAUSE PERSONAL INJURY OR DEATH AND YOU AGREE\nTHAT YOU ARE FULLY RESPONSIBLE FOR ANY CLAIMS, COSTS, DAMAGES, EXPENSES, AND\nATTORNEYS' FEES ARISING OUT OF ANY SUCH USE, EVEN IF ANY CLAIM ALLEGES THAT\nINTEL WAS NEGLIGENT REGARDING THE DESIGN OR MANUFACTURE OF THE SOFTWARE.\n\nLIMITATION OF LIABILITY. IN NO EVENT WILL INTEL BE LIABLE FOR ANY DIRECT,\nINDIRECT, INCIDENTAL, SPECIAL, EXEMPLARY, OR CONSEQUENTIAL DAMAGES (INCLUDING,\nBUT NOT LIMITED TO, PROCUREMENT OF SUBSTITUTE GOODS OR SERVICES; LOSS OF USE,\nDATA, OR PROFITS; OR BUSINESS INTERRUPTION) HOWEVER CAUSED AND ON ANY THEORY OF\nLIABILITY, WHETHER IN CONTRACT, STRICT LIABILITY, OR TORT (INCLUDING NEGLIGENCE\nOR OTHERWISE) ARISING IN ANY WAY OUT OF THE USE OF THIS SOFTWARE, EVEN IF\nADVISED OF THE POSSIBILITY OF SUCH DAMAGE.\n\nNo support. Intel may make changes to the Software, at any time without notice,\nand is not obligated to support, update or provide training for the Software. \n\nTermination. Your right to use the Software is terminated in the event of your\nbreach of this license.\n\nFeedback. Should you provide Intel with comments, modifications, corrections,\nenhancements or other input (\"Feedback\") related to the Software, Intel will be\nfree to use, disclose, reproduce, license or otherwise distribute or exploit the\nFeedback in its sole discretion without any obligations or restrictions of any\nkind, including without limitation, intellectual property rights or licensing\nobligations.\n\nCompliance with laws. You agree to comply with all relevant laws and regulations\ngoverning your use, transfer, import or export (or prohibition thereof) of the\nSoftware.\n\nGoverning law. All disputes will be governed by the laws of the United States of\nAmerica and the State of Delaware without reference to conflict of law\nprinciples and subject to the exclusive jurisdiction of the state or federal\ncourts sitting in the State of Delaware, and each party agrees that it submits\nto the personal jurisdiction and venue of those courts and waives any\nobjections. THE UNITED NATIONS CONVENTION ON CONTRACTS FOR THE INTERNATIONAL\nSALE OF GOODS (1980) IS SPECIFICALLY EXCLUDED AND WILL NOT APPLY TO THE SOFTWARE.\n\nmscr-chi_table_LICENSE.txt:\n\n                          License Agreement\n                          For chi_table.h\n\nCopyright (C) 2007 Per-Erik Forssen, all rights reserved.\n\nRedistribution and use in source and binary forms, with or without modification,\nare permitted provided that the following conditions are met:\n\n  * Redistribution's of source code must retain the above copyright notice,\n    this list of conditions and the following disclaimer.\n\n  * Redistribution's in binary form must reproduce the above copyright notice,\n    this list of conditions and the following disclaimer in the documentation\n    and/or other materials provided with the distribution.\n\n  * The name of the copyright holders may not be used to endorse or promote products\n    derived from this software without specific prior written permission.\n\nThis software is provided by the copyright holders and contributors \"as is\" and\nany express or implied warranties, including, but not limited to, the implied\nwarranties of merchantability and fitness for a particular purpose are disclaimed.\nIn no event shall the Intel Corporation or contributors be liable for any direct,\nindirect, incidental, special, exemplary, or consequential damages\n(including, but not limited to, procurement of substitute goods or services;\nloss of use, data, or profits; or business interruption) however caused\nand on any theory of liability, whether in contract, strict liability,\nor tort (including negligence or otherwise) arising in any way out of\nthe use of this software, even if advised of the possibility of such damage."  # Fixed Up OpenCV4
  w21 = string[] ["averaging_quaternions - https://github.com/tolgabirdal/averaging_quaternions\n\nThe MIT License (MIT)\n\nCopyright (c) 2014 Tolga Birdal\n\nPermission is hereby granted, free of charge, to any person obtaining a copy\nof this software and associated documentation files (the \"Software\"), to deal\nin the Software without restriction, including without limitation the rights\nto use, copy, modify, merge, publish, distribute, sublicense, and/or sell\ncopies of the Software, and to permit persons to whom the Software is\nfurnished to do so, subject to the following conditions:\n\nThe above copyright notice and this permission notice shall be included in all\ncopies or substantial portions of the Software.\n\nTHE SOFTWARE IS PROVIDED \"AS IS\", WITHOUT WARRANTY OF ANY KIND, EXPRESS OR\nIMPLIED, INCLUDING BUT NOT LIMITED TO THE WARRANTIES OF MERCHANTABILITY,\nFITNESS FOR A PARTICULAR PURPOSE AND NONINFRINGEMENT. IN NO EVENT SHALL THE\nAUTHORS OR COPYRIGHT HOLDERS BE LIABLE FOR ANY CLAIM, DAMAGES OR OTHER\nLIABILITY, WHETHER IN AN ACTION OF CONTRACT, TORT OR OTHERWISE, ARISING FROM,\nOUT OF OR IN CONNECTION WITH THE SOFTWARE OR THE USE OR OTHER DEALINGS IN THE\nSOFTWARE.", "Spot Model - https://www.cs.cmu.edu/~kmcrane/Projects/ModelRepository/ \n\nCC0 1.0 Universal", "ROS 2 Windows Media Foundation Camera Driver - https//:github.com/ms-iot/ros_msft_camera\n\nCopyright (C) Microsoft Corporation. All rights reserved.\n\nReleased under the MIT Licence\nPermission is hereby granted, free of charge, to any person obtaining a copy\nof this software and associated documentation files (the \"Software\"), to deal\nin the Software without restriction, including without limitation the rights\nto use, copy, modify, merge, publish, distribute, sublicense, and/or sell\ncopies of the Software, and to permit persons to whom the Software is\nfurnished to do so, subject to the following conditions:\n\nThe above copyright notice and this permission notice shall be included in all\ncopies or substantial portions of the Software.\n\nTHE SOFTWARE IS PROVIDED \"AS IS\", WITHOUT WARRANTY OF ANY KIND, EXPRESS OR\nIMPLIED, INCLUDING BUT NOT LIMITED TO THE WARRANTIES OF MERCHANTABILITY,\nFITNESS FOR A PARTICULAR PURPOSE AND NONINFRINGEMENT. IN NO EVENT SHALL THE\nAUTHORS OR COPYRIGHT HOLDERS BE LIABLE FOR ANY CLAIM, DAMAGES OR OTHER\nLIABILITY, WHETHER IN AN ACTION OF CONTRACT, TORT OR OTHERWISE, ARISING FROM,\nOUT OF OR IN CONNECTION WITH THE SOFTWARE OR THE USE OR OTHER DEALINGS IN THE\nSOFTWARE."]  # Additional
  w25 = map{string, string} {}  # Size: 0
  w26 = cluster{"name":string, string}[] [{"name"="abseil", "Abseil - https://abseil.io/"}, {"name"="apriltag", "AprilTag - https://april.eecs.umich.edu/software/apriltag"}, {"name"="eigen3", "Eigen - https://eigen.tuxfamily.org/index.php"}, {"name"="flatbuffers", "flatbuffers - https://github.com/google/flatbuffers"}, {"name"="libaec", "labaec - https://gitlab.dkrz.de/k202009/libaec"}, {"name"="libjpeg-turbo", "libjpeg-turbo - https://libjpeg-turbo.org/"}, {"name"="liblzma", "XZ Utils - https://github.com/tukaani-project/xz"}, {"name"="libpng", "libpng - https://www.libpng.org/pub/png/libpng.html"}, {"name"="libwebp", "libwebp - https://chromium.googlesource.com/webm/libwebp"}, {"name"="opencv4", "Opencv - https://opencv.org"}, {"name"="protobuf", "Protocol Buffers - https://protobuf.dev/"}, {"name"="pthreads", "PThreads4w - https://sourceforge.net/projects/pthreads4w/"}, {"name"="tiff", "libtiff - https://libtiff.gitlab.io/libtiff/"}, {"name"="tinyobjloader", "tinyobjloader - https://github.com/tinyobjloader/tinyobjloader"}, {"name"="utf8-range", "utf8-range - https://github.com/protocolbuffers/protobuf"}, {"name"="zlib", "Zlib - https://www.zlib.net/"}, {"name"="bzip2", "bzip2 - https://sourceware.org/bzip2/"}, {"name"="curl", "curl - https://curl.se/"}, {"name"="giflib", "giflib - https://giflib.sourceforge.net/"}, {"name"="hdf5", "HDF5 - https://github.com/HDFGroup/hdf5"}, {"name"="leptonica", "Leptonica - http://www.leptonica.org/"}, {"name"="libarchive", "libarchive - https://www.libarchive.org/"}, {"name"="libxml2", "libxml2 - https://gitlab.gnome.org/GNOME/libxml2"}, {"name"="lz4", "lz4 - https://github.com/lz4/lz4 "}, {"name"="openjpeg", "OpenJPEG - https://www.openjpeg.org/"}, {"name"="openssl", "OpenSSL - https://www.openssl.org/"}, {"name"="tesseract", "Tesseract OCR - https://github.com/tesseract-ocr/tesseract"}, {"name"="nu-book-zxing-cpp", "ZXing-C++ - https://github.com/zxing-cpp/zxing-cpp"}, {"name"="ffmpeg", "FFmpeg - https://www.ffmpeg.org/"}]  # Additional info
  n1 = for {
    tunnel: w26 -> [w32] mode=indexing
    shift-right: [w29] -> w24
    shift-left: w25 -> [w28]
    n2 = Unbundle(w32) -> ("name"=w31:string, w30:string)
    n3 = Insert Into Map(map in=w28, key=w31, value=w30) -> (map out=w29:map{string, string})  [unwired: 2 out]
  }
  n4 = call <vilib>:"Recursive File List.vi"("pattern"="copyright", "Folder Path"="Folder Path") -> ("All Files in Dir"=w27:path[])  [unwired: 5 in, 4 out]
  n5 = for {
    tunnel: w27 -> [w40] mode=indexing
    tunnel: [w38] -> w8 mode=indexing if=w37
    tunnel: w24 -> [w39]
    shift-right: [w36] -> _
    shift-left: w5 -> [w35]
    tunnel: [w34] -> w3 mode=indexing if=w33
    n6 = Strip Path(path=w40) -> (stripped path=w41:path, name=w42:string)
    n7 = case shown="\"copyright\"" w42 {
      tunnel: w41 -> [_ w51]
      tunnel: w40 -> [_ w53]
      tunnel: w39 -> [_ w52]
      tunnel: [_ w49] -> w38
      tunnel: [_ w48] -> w37
      tunnel: [w43 w47] -> w36
      tunnel: w35 -> [w43 w46]
      tunnel: [_ w45] -> w34
      tunnel: [_ w44] -> w33
      frame Default {
      }
      frame "copyright" {
        n8 = Strip Path(path=w51) -> (name=w50:string)  [unwired: 1 out]
        n9 = case shown="Default" w50 {
          selector: w50 -> [_ w59]
          tunnel: w53 -> [_ w73]
          tunnel: w52 -> [_ w68]
          tunnel: [_ w66] -> w49
          tunnel: [_ w57] -> w48
          tunnel: [w54 w64] -> w47
          tunnel: w46 -> [w54 w65]
          tunnel: [_ w58] -> w45
          tunnel: [_ w56] -> w44
          frame "libiconv", "opencv4", "zstd" {
          }
          frame Default {
            n10 = Match Pattern(string=w59, regular expression="^boost-") -> (offset past match=w60:i32)  [unwired: 1 in, 3 out]
            n11 = case shown="Default" w60 {
              tunnel: ["boost" w75] -> w58
              tunnel: w59 -> [_ w75]
              frame Default {
              }
              frame -1 {
              }
            }
            n12 = Read from Text File(file (use dialog)=w73) -> (text=w72:string)  [unwired: 3 in, 3 out]
            n13 = Look In Map(map=w68, key=w58) -> (key not found?=w56:bool, value=w67:string)  [unwired: 1 in]
            n14 = call <vilib>:"Trim Whitespace.vi"("string"=w72) -> ("trimmed string"=w69:string)  [unwired: 1 in]
            n15 = Insert Into Set(10:w58, 11:w65) -> (2:w63:bool, 3:w64:set{string})
            n16 = Not(x=w56) -> (.not. x?=w55:bool)
            n17 = Not(x=w63) -> (.not. x?=w62:bool)
            n18 = And(x=w55, y=w62) -> (x .and. y?=w57:bool)
            n19 = Format Into String(format string="%s\n\n%s", w67, w69) -> (resulting string=w71:string)  [unwired: 2 in, 1 out]
            n20 = call <vilib>:"Trim Whitespace.vi"("string"=w71) -> ("trimmed string"=w66:string)  [unwired: 1 in]
          }
        }
      }
    }
  }
  n21 = call <vilib>:"Application Directory.vi"() -> ("Application Directory"=w18:path)
  n22 = Build Array (concatenate)(w4, w20, w7, w6, w8, w21) -> (w22:string[])
  n23 = call "Remove Duplicates From 1D Array.vim"("array"=w3) -> ("array with duplicates removed"=→"Missing Entires":string[])  [unwired: 10 in]
  n24 = Build Path(base path=w18, name or relative path=path "common/bin/COPYING") -> (appended path=w16:path)
  n25 = call <vilib>:"1D String Array to Delimited String.vi"("delimiter"="\n\n----------------------------------\n\n" ("string"), "string array"=w22) -> ("delimited string"=w10:string)  [unwired: 9 in]
  n26 = Open/Create/Replace File(file path (use dialog)=w16, operation (0:open)=T1."replace or create") -> (refnum out=w13:refnum<file>, error out=w14:errorcluster)  [unwired: 4 in, 1 out]
  n27 = Write to Text File(file (use dialog)=w13, text=w10, error in=w14) -> (refnum out=w11:refnum<file>, error out=w12:errorcluster)  [unwired: 1 in, 1 out]
  n28 = Close File(refnum=w11, error in=w12) -> (error out=→"error out":errorcluster)  [unwired: 1 out]
